vi "Normalize.vi"(8 "error in":errorcluster, 11 "Vec3d in":refnum<class "Vec3d Class.lvclass">) -> (0 "error out":errorcluster, 3 "Vec3d out":refnum<class "Vec3d Class.lvclass">)   [LabVIEW 2011, in "Vec3d Class.lvclass"]
uses:
  Vec3d Class.lvclass
  Vec3d Class.lvclass/Vec3d Class.ctl
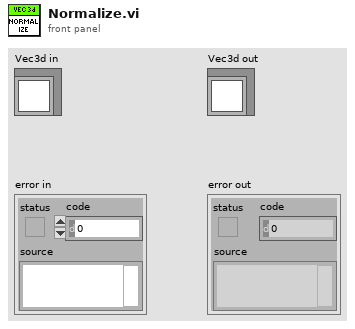
[diagram p1: front panel]
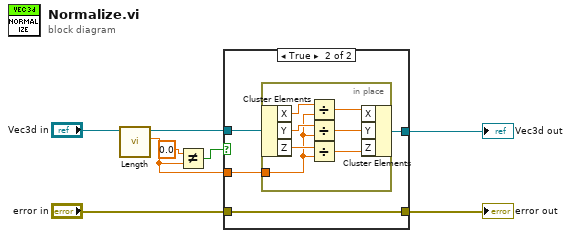
[diagram p0: block diagram]
diagram:
  n1 = call-dynamic "Length.vi"("Vec3d in"="Vec3d in") -> ("Length"=w4:dbl, "Vec3d out"=w6:refnum<class "Vec3d Class.lvclass">)  [unwired: 8 in, 1 out]
  n2 = Not Equal?(x=0.0, y=w4) -> (x != y?=w5:bool)
  n3 = case shown="True" w5 {
    tunnel: [w10 w14] -> w7
    tunnel: w6 -> [w10 w13]
    tunnel: w4 -> [_ w12]
    tunnel: "error in" -> [w9 w11]
    tunnel: [w9 w11] -> w1
    frame False {
      # "Don't attempt to normalize\nzero vector"
    }
    frame True {
      n4 = in-place {
        in-place-border: w12 -> [w18]
        n5 = in-place-cluster #1(w13) -> ("X"=w21:dbl, "Y"=w20:dbl, "Z"=w19:dbl)
        n6 = Divide(x=w21, y=w18) -> (x/y=w17:dbl)
        n7 = Divide(x=w20, y=w18) -> (x/y=w16:dbl)
        n8 = Divide(x=w19, y=w18) -> (x/y=w15:dbl)
        n9 = in-place-cluster #1("X"=w17, "Y"=w16, "Z"=w15) -> (w14:refnum<class "Vec3d Class.lvclass">)
      }
    }
  }
  "error out" <- w1
  "Vec3d out" <- w7
